vi "Set-to-startup-condition.vi"(8 "error in (no error)":errorcluster, 11 "Panes in":T1) -> (0 "error out":errorcluster, 3 "Panes out":T1)   [LabVIEW 2013, in "CameraVision.lvlib" / "CV-Panes.lvclass"]
uses:
  CV-Panes.lvclass
  Object-reference.ctl
  CV-Panes.lvclass/CV-Panes.ctl
  Read-Panes.vi
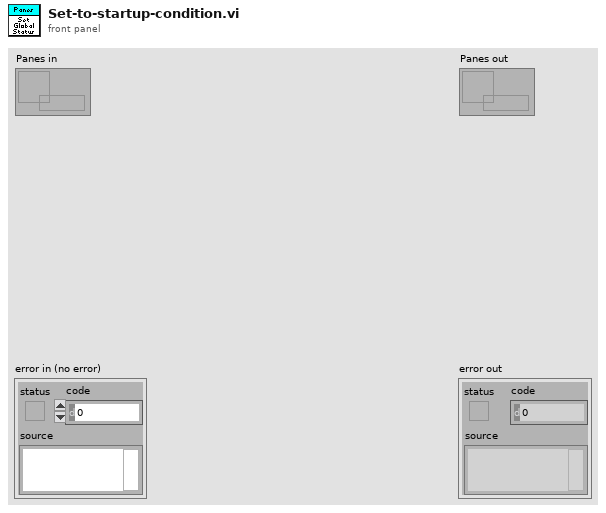
[diagram p1: front panel]
types:
  T1 = typedef "CameraVision.lvlib/CV-Panes.lvclass/Object-reference.ctl" = refnum<data-value>
  T2 = typedef "CV-Panes.lvclass/Pane-settings.ctl" = cluster{"Pane-name":T3, "Startup visible?":bool, "Currently visible?":bool, "Splitters":T4[], "Pane-reference":refnum<vi>}
  T3 = typedef "CV-Panes.lvclass/Pane-names.ctl" = enum16{"Toolbar", "Help bar", "Toolbar lower border", "Settings", "Displays", "Status bar upper border", "General state bar", "Information bar"}
  T4 = typedef "CV-Panes.lvclass/Splitter-settings.ctl" = cluster{"Splitter-name":T5, "Position shown":i32, "Position hidden":i32, "Splitter reference":refnum<vi>}
  T5 = typedef "CV-Panes.lvclass/Splitter-names.ctl" = enum16{"Upper toolbar splitter", "Help bar splitter", "Lower toolbar splitter", "Upper status bar splitter", "Lower status bar splitter", "Splitter", "Settings splitter"}
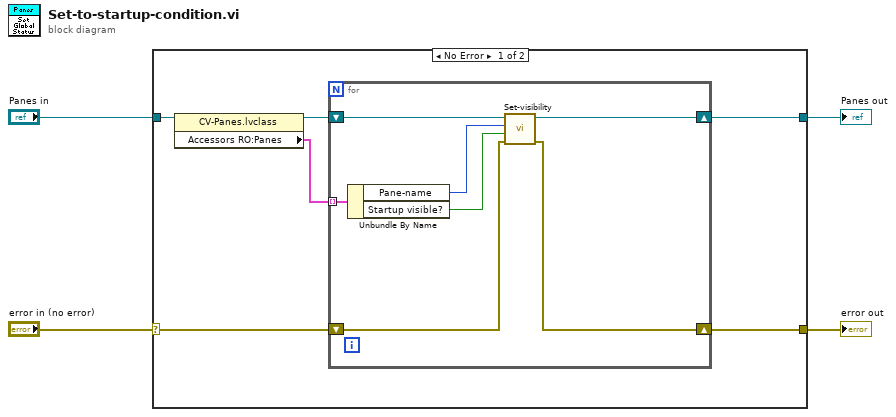
[diagram p0: block diagram]
diagram:
  n1 = case shown="No Error" "error in (no error)" {
    selector: "error in (no error)" -> [w7 w18]
    tunnel: [w5 w18] -> w3
    tunnel: [w6 w19] -> w1
    tunnel: "Panes in" -> [w10 w19]
    frame No Error {
      n2 = property class="CV-Panes.lvclass"(reference=w10) -> (reference out=w9:T1, "Accessors RO:Panes"=w8:T2[])  [unwired: 1 in, 1 out]
      n3 = for {
        shift-right: [w11] -> w6
        shift-left: w9 -> [w16]
        tunnel: w8 -> [w17] mode=indexing
        shift-right: [w12] -> w5
        shift-left: w7 -> [w13]
        n4 = Unbundle By Name(w17) -> ("Pane-name"=w15:T3, "Startup visible?"=w14:bool)
        n5 = call "Set-visibility.vi"("error in (no error)"=w13, "Visibility"=w14, "Pane"=w15, "Panes in"=w16) -> ("error out"=w12:errorcluster, "Panes out"=w11:T1)  [unwired: 6 in]
      }
    }
    frame Error {
    }
  }
  "error out" <- w3
  "Panes out" <- w1
